vi "이효재_Car Wash.vi"() -> ()   [LabVIEW 2018]
uses:
  Controls/Car Wash Indicators.ctl
  Controls/Wash Options.ctl
panel:
  in  "시작":bool
  out "경과 시간(초)":dbl format="%0.2f"
  in  "stop":bool
  out "세차기 입구":bool
  in  "세차 옵션":T1
  in  "자동차 위치 슬라이더":u8(slide) max=3 scale=0.0..4.0
  out "세차 인디케이터":T2
  # "입구 콘솔"
  # "세차 디스플레이"
  # "자동차 위치 시뮬레이션"
  # "애벌 세차\n고압 세차\n저압 왁스\n얼룩 제거 린스"
  # "자동차 바닥 세차\n벌레 제거"
  # "타이어 광택\n공기 건조"
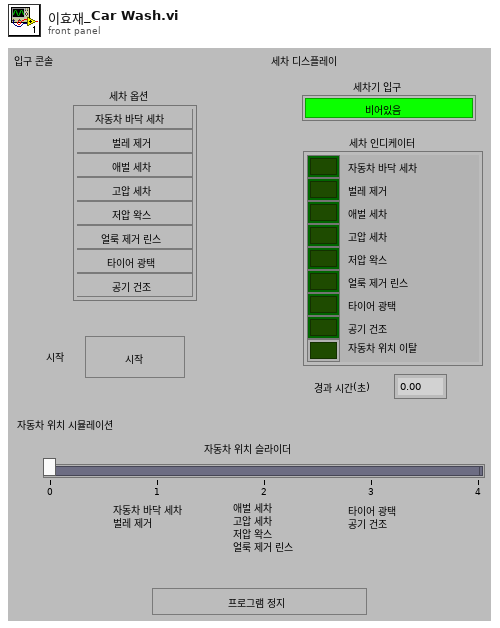
[diagram p1: front panel]
types:
  T1 = typedef "Wash Options.ctl" = cluster{"자동차 바닥 세차":bool, "벌레 제거":bool, "애벌 세차":bool, "고압 세차":bool, "저압 왁스":bool, "얼룩 제거 린스":bool, "타이어 광택":bool, "공기 건조":bool}
  T2 = typedef "Car Wash Indicators.ctl" = cluster{"자동차 바닥 세차":bool, "벌레 제거":bool, "애벌 세차":bool, "고압 세차":bool, "저압 왁스":bool, "얼룩 제거 린스":bool, "타이어 광택":bool, "공기 건조":bool, "자동차 위치 이탈":bool}
  T3 = enum8{"Enabled", "Disabled", "Disabled and Grayed Out"}
  T4 = enum16{"자동차", "国饭", "局国", "고압", "저압", "얼룩", "타이어", "공기"}[]
  T5 = enum16{"자동차", "国饭", "局国", "고압", "저압", "얼룩", "타이어", "공기"}
  T6 = cluster{"Value[0]":bool, "Value[1]":bool, "Value[2]":bool, "Value[3]":bool, "Value[4]":bool, "Value[5]":bool, "Value[6]":bool, "Value[7]":bool, "Value[8]":bool}
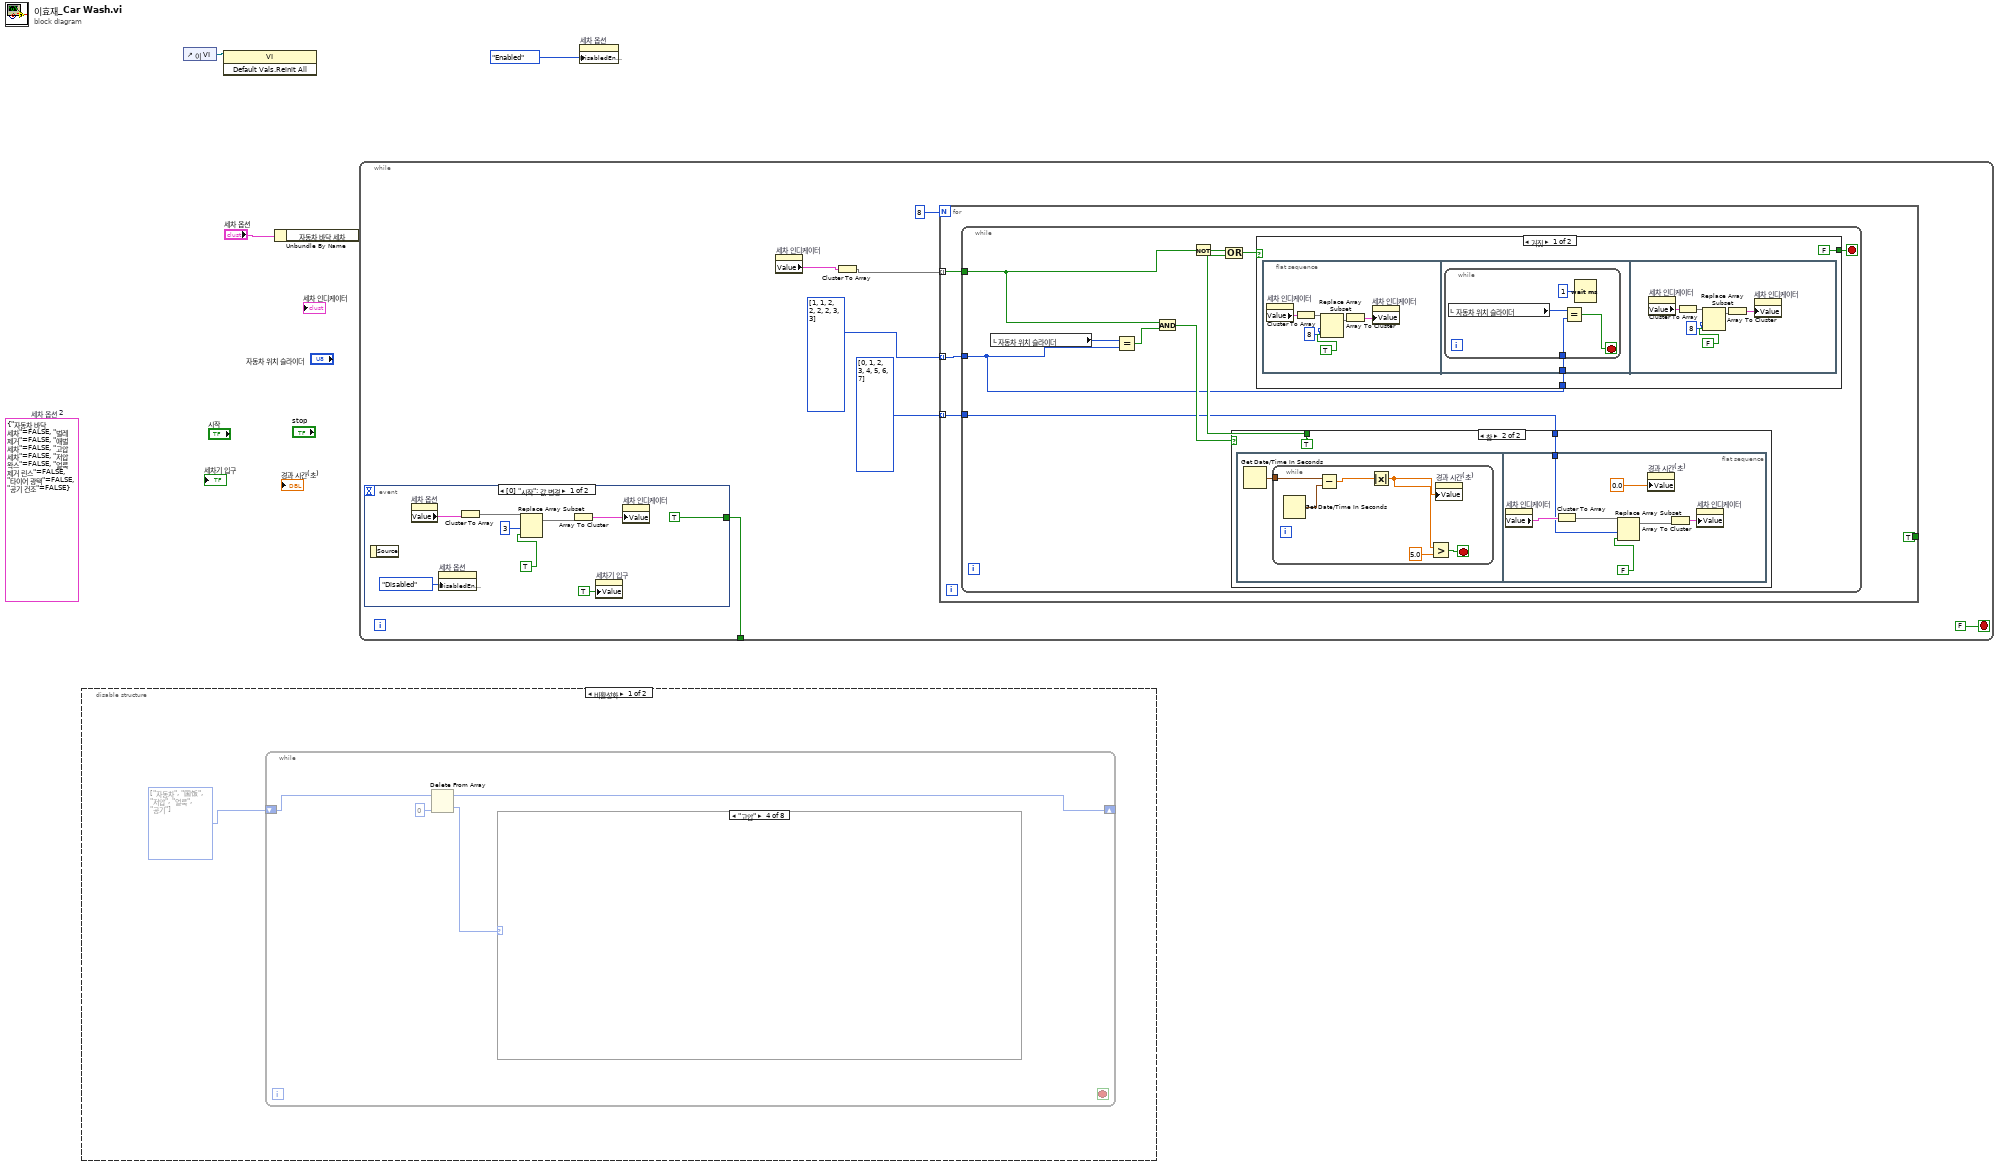
[diagram p0: block diagram]
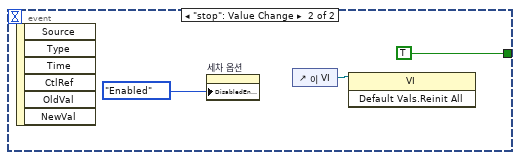
[diagram p12: hidden frame]
diagram:
  (unwired) T1 {"자동차 바닥 세차"=FALSE, "벌레 제거"=FALSE, "애벌 세차"=FALSE, "고압 세차"=FALSE, "저압 왁스"=FALSE, "얼룩 제거 린스"=FALSE, "타이어 광택"=FALSE, "공기 건조"=FALSE}  # 세차 옵션 2
  n1 = disable-structure shown="비활성화" {
    frame Disabled {
      w4 = T4 [enum."자동차", enum."国饭", enum."저압", enum."얼룩", enum."공기"] items=["자동차", "国饭", "局国", "고압", "저압", "얼룩", "타이어", "공기"]
      n2 = while {
        shift-right: [w7] -> _
        shift-left: w4 -> [w6]
        stop <- _ stop-if-true
        n3 = Delete From Array(array=w6, index=0 ("인덱스")) -> (deleted portion=w8:T5, array with subset deleted=w7:T4)  [unwired: 1 in]
        n4 = case shown="\"고압\"" w8 {
          frame "자동차", Default {
          }
          frame "国饭" {
          }
          frame "局国" {
          }
          frame "고압" {
          }
          frame "저압" {
          }
          frame "얼룩" {
          }
          frame "타이어" {
          }
          frame "공기" {
          }
        }
      }
    }
    frame Enabled {
    }
  }
  n5 = control-ref of="이 VI"() -> (w2:refnum<vi>)
  n6 = invoke class="VI" method="Default Vals.Reinit All"(reference=w2) -> ()  [unwired: 2 in, 3 out]
  n7 = Unbundle By Name("세차 옵션") -> ()  [unwired: 1 out]
  n8 = while {
    tunnel: [w14] -> _
    stop <- FALSE stop-if-true
    n9 = event shown="[0] \"시작\": 값 변경" {
      selector: _ -> [_ _]
      dyn-events: _ -> [_ _]
      timeout: _ -> [_ _]
      tunnel: [TRUE TRUE] -> w14
      event "시작": Value Change {
        n10 = event-data() -> ()  [unwired: 1 in, 1 out]
        n11 = property on="세차 옵션" class="Clust (엄격한)"() -> ("Value"=w74:T1)  [unwired: 2 in, 2 out]
        n12 = property on="세차 옵션" class="Clust (엄격한)"("DisabledEnum"=T3."Disabled" ("비활성화")) -> ()  [unwired: 2 in, 2 out]
        n13 = Cluster To Array(cluster=w74) -> (array=w75:bool[])
        n14 = Replace Array Subset(array=w75, new element=TRUE ("새 원소/부분배열"), index=3 ("인덱스")) -> (w72:bool[])
        n15 = Array To Cluster(array=w72) -> (cluster=w73:T6)
        n16 = property on="세차기 입구" class="Bool (엄격한)"("Value"=TRUE ("세차기 입구")) -> ()  [unwired: 2 in, 2 out]
        n17 = property on="세차 인디케이터" class="Clust (엄격한)"("Value"=w73) -> ()  [unwired: 2 in, 2 out]
      }
      event "stop": Value Change {
        n18 = event-data() -> ()  [unwired: 1 in, 6 out]
        n19 = property on="세차 옵션" class="Clust (엄격한)"("DisabledEnum"=T3."Enabled" ("비활성화")) -> ()  [unwired: 2 in, 2 out]
        n20 = control-ref of="이 VI"() -> (w78:refnum<vi>)
        n21 = invoke class="VI" method="Default Vals.Reinit All"(reference=w78) -> ()  [unwired: 2 in, 3 out]
      }
    }
    n22 = property on="세차 인디케이터" class="Clust (엄격한)"() -> ("Value"=w13:T2)  [unwired: 2 in, 2 out]
    n23 = Cluster To Array(cluster=w13) -> (array=w12:bool[])
    n24 = for {
      N: 8 -> [_]
      tunnel: w12 -> [w19] mode=indexing
      tunnel: i32[] [0, 1, 2, 3, 4, 5, 6, 7] -> [w17] mode=indexing
      tunnel: i32[] [1, 1, 2, 2, 2, 2, 3, 3] -> [w18] mode=indexing
      tunnel: [TRUE] -> _
      n25 = while {
        tunnel: w19 -> [w23]
        tunnel: w18 -> [w20]
        tunnel: w17 -> [w21]
        stop <- w22 stop-if-true
        n26 = local read "자동차 위치 슬라이더"() -> (w28:u8)
        n27 = Equal?(x=w28, y=w20) -> (x = y?=w27:bool)
        n28 = And(x=w23, y=w27) -> (x .and. y?=w25:bool)
        n29 = Not(x=w23) -> (.not. x?=w29:bool)
        n30 = case shown="참" w25 {
          selector: w25 -> [w30 _]
          tunnel: [w30 TRUE] -> w24
          tunnel: w21 -> [_ w31]
          frame False {
          }
          frame True {
            n31 = flat-sequence {
              tunnel: w31 -> [w40]
              frame #0 {
                n32 = Get Date/Time In Seconds() -> (seconds since 1Jan1904=w33:timestamp)
                n33 = while {
                  tunnel: w33 -> [w39]
                  stop <- w36 stop-if-true
                  n34 = Get Date/Time In Seconds() -> (seconds since 1Jan1904=w38:timestamp)
                  n35 = Subtract(x=w39, y=w38) -> (x-y=w37:dbl)
                  n36 = Absolute Value(x=w37) -> (abs(x)=w34:dbl)
                  n37 = Greater?(x=w34, y=5.0) -> (0:w36:bool)
                  n38 = property on="경과 시간(초)" class="DigNum (엄격한)"("Value"=w34) -> ()  [unwired: 2 in, 2 out]
                }
              }
              frame #1 {
                n39 = property on="세차 인디케이터" class="Clust (엄격한)"() -> ("Value"=w44:T2)  [unwired: 2 in, 2 out]
                n40 = Cluster To Array(cluster=w44) -> (array=w42:bool[])
                n41 = Replace Array Subset(array=w42, new element=FALSE ("새 원소/부분배열"), index=w40) -> (w43:bool[])
                n42 = property on="경과 시간(초)" class="DigNum (엄격한)"("Value"=0.0 ("경과 시간(초)")) -> ()  [unwired: 2 in, 2 out]
                n43 = Array To Cluster(array=w43) -> (cluster=w45:T6)
                n44 = property on="세차 인디케이터" class="Clust (엄격한)"("Value"=w45) -> ()  [unwired: 2 in, 2 out]
              }
            }
          }
        }
        n45 = Compound Arithmetic op=OR ("복합 연산")(w29, w24) -> (w26:bool)
        n46 = case shown="거짓" w26 {
          selector: w26 -> [_ w66]
          tunnel: [FALSE w66] -> w22
          tunnel: w20 -> [w47 _]
          frame False {
            n47 = flat-sequence {
              tunnel: w47 -> [w55]
              frame #0 {
                n48 = property on="세차 인디케이터" class="Clust (엄격한)"() -> ("Value"=w52:T2)  [unwired: 2 in, 2 out]
                n49 = Cluster To Array(cluster=w52) -> (array=w54:bool[])
                n50 = Replace Array Subset(array=w54, new element=TRUE ("새 원소/부분배열"), index=8 ("인덱스")) -> (w53:bool[])
                n51 = Array To Cluster(array=w53) -> (cluster=w51:T6)
                n52 = property on="세차 인디케이터" class="Clust (엄격한)"("Value"=w51) -> ()  [unwired: 2 in, 2 out]
              }
              frame #1 {
                n53 = while {
                  tunnel: w55 -> [w56]
                  stop <- w58 stop-if-true
                  n54 = local read "자동차 위치 슬라이더"() -> (w59:u8)
                  n55 = Equal?(x=w59, y=w56) -> (x = y?=w58:bool)
                  n56 = Wait (ms)(milliseconds to wait=u32 1 ("대기 시간 (ms)")) -> ()  [unwired: 1 out]
                }
              }
              frame #2 {
                n57 = property on="세차 인디케이터" class="Clust (엄격한)"() -> ("Value"=w63:T2)  [unwired: 2 in, 2 out]
                n58 = Cluster To Array(cluster=w63) -> (array=w65:bool[])
                n59 = Replace Array Subset(array=w65, new element=FALSE ("새 원소/부분배열"), index=8 ("인덱스")) -> (w64:bool[])
                n60 = Array To Cluster(array=w64) -> (cluster=w62:T6)
                n61 = property on="세차 인디케이터" class="Clust (엄격한)"("Value"=w62) -> ()  [unwired: 2 in, 2 out]
              }
            }
          }
          frame True {
          }
        }
      }
    }
  }
  n62 = property on="세차 옵션" class="Clust (엄격한)"("DisabledEnum"=T3."Enabled" ("비활성화")) -> ()  [unwired: 2 in, 2 out]
